vi "TOOLweb ALLE DATEN.vi"(4 "error in (no error)":errorcluster caption="Fehler (Eingang, kein Fehler)", 5 "IP-Adresse (localhost)":string="127.0.0.1", 7 "Anzahl Gase":i32=18) -> (0 "error out":errorcluster caption="Fehler (Ausgang)", 1 "Diagnose":T1, 2 "Info":T3, 3 "Signalverläufe":T2)   [LabVIEW 2020, in "FT-IR.lvlib" / "TOOLweb Interface.lvlib"]
doc: "Holt mit einer HTTP-POST-Anforderung gemäß TOOLweb-Protokoll Messdaten, Einstellungen und Diagnose-Information vom MKS MultiGas 2030 Analyzer. Alle Daten werden zeitsparend in einem einzigen Poll Request zusammengefasst, damit nur einmal eine TCP/IP-Verbindung geöffnet werden muss.\n\nAlle Ergebnis-Datentypen sind als Typdefinitionen in der Bibliothek \"Datentypen\" enthalten\" und erlauben so eine spätere Erweiterung.\n\nFalls \"Anzahl Gase\" unverbunden bleibt, wird der Standardwert 18 verwendet.\n \nFalls der TOOLWeb-Server nicht auf demselben Rechner arbeitet, kann mit \"IP-Adresse\" eine beliebiger Host adressiert werden. Ein unverbundener Eingang spricht den lokalen Host an."
uses:
  TOOLweb Interface.lvlib
  TOOLweb Interface Hilfs-VIs.lvlib
  TOOLweb Info.ctl
  Typdefinitionen.lvlib
  TOOLweb Diagnose.ctl
  TOOLweb Signalverlaeufe.ctl
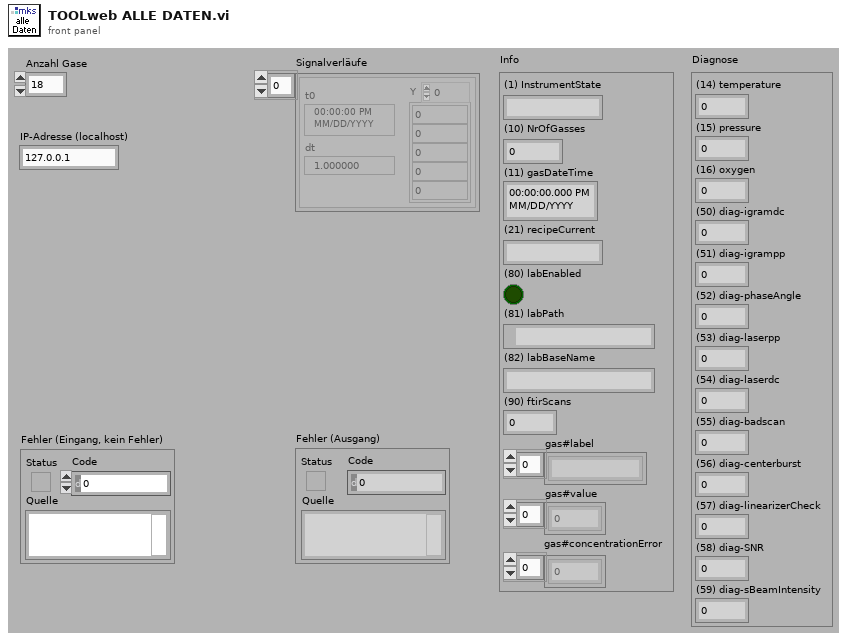
[diagram p1: front panel]
types:
  T1 = typedef "FT-IR.lvlib/TOOLweb Interface.lvlib/Typdefinitionen.lvlib/TOOLweb Diagnose.ctl" = cluster{"(14) temperature":sgl, "(15) pressure":sgl, "(16) oxygen":sgl, "(50) diag-igramdc":sgl, "(51) diag-igrampp":sgl, "(52) diag-phaseAngle":sgl, "(53) diag-laserpp":sgl, "(54) diag-laserdc":sgl, "(55) diag-badscan":sgl, "(56) diag-centerburst":sgl, "(57) diag-linearizerCheck":sgl, "(58) diag-SNR":sgl, "(59) diag-sBeamIntensity":sgl}
  T2 = typedef "FT-IR.lvlib/TOOLweb Interface.lvlib/Typdefinitionen.lvlib/TOOLweb Signalverlaeufe.ctl" = waveform(dbl)[]
  T3 = typedef "FT-IR.lvlib/TOOLweb Interface.lvlib/Typdefinitionen.lvlib/TOOLweb Info.ctl" = cluster{"(1) InstrumentState":string, "(10) NrOfGasses":i32, "(11) gasDateTime":timestamp, "(21) recipeCurrent":string, "(80) labEnabled":bool, "(81) labPath":path, "(82) labBaseName":string, "(90) ftirScans":i32, "gas#label":string[], "gas#value":dbl[], "gas#concentrationError":dbl[]}
  T4 = cluster{"(1) InstrumentState":string, "(10) NrOfGasses":dbl, "(11) gasDateTime":timestamp, "(21) recipeCurrent":string, "(80) labEnabled":bool, "(81) labPath":path, "(82) labBaseName":string, "(90) ftirScans":i32, "gas#label":string[], "gas#value":dbl[], "gas#concentrationError":dbl[]}
  T5 = cluster{"(14) temperature":dbl, "(15) pressure":dbl, "(16) oxygen":dbl, "(50) diag-igramdc":dbl, "(51) diag-igrampp":dbl, "(52) diag-phaseAngle":dbl, "(53) diag-laserpp":dbl, "(54) diag-laserdc":dbl, "(55) diag-badscan":dbl, "(56) diag-centerburst":dbl, "(57) diag-linearizerCheck":dbl, "(58) diag-SNR":dbl, "(59) diag-sBeamIntensity":dbl}
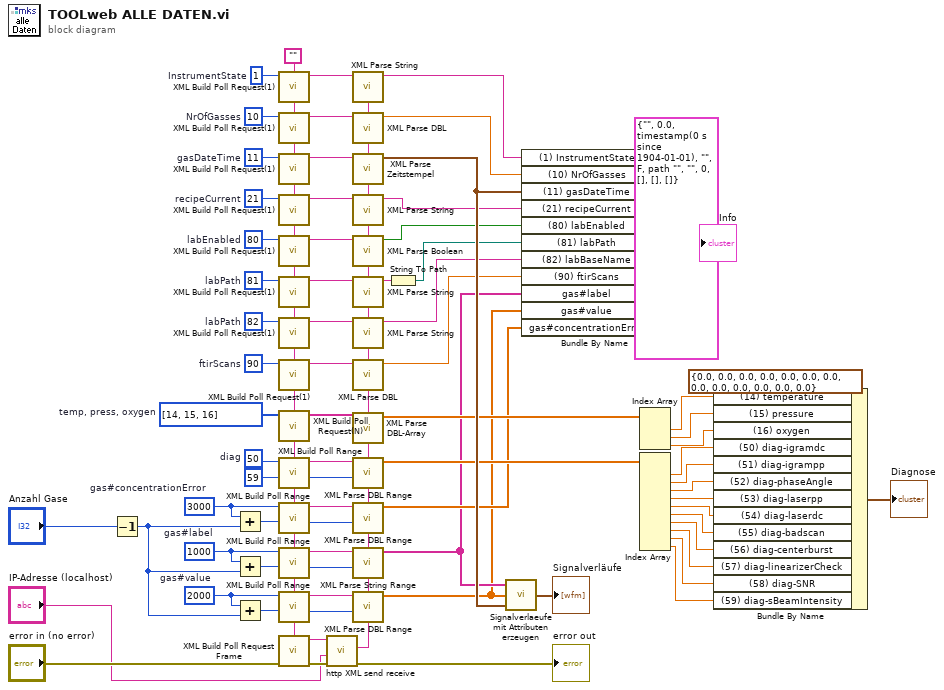
[diagram p0: block diagram]
diagram:
  w33 = 90  # ftirScans
  w37 = 82  # labPath
  w43 = 81  # labPath
  w61 = 50  # diag
  w74 = 1  # InstrumentState
  w76 = 3000  # gas#concentrationError
  w88 = i32[] [14, 15, 16]  # temp, press, oxygen
  w92 = 80  # labEnabled
  w93 = 21  # recipeCurrent
  w94 = 10  # NrOfGasses
  w97 = 2000  # gas#value
  w98 = 1000  # gas#label
  w99 = 11  # gasDateTime
  n1 = Decrement(x="Anzahl Gase") -> (x-1=w75:i32)
  n2 = Add(x=w76, y=w75) -> (x+y=w77:i32)
  n3 = Add(x=w98, y=w75) -> (x+y=w90:i32)
  n4 = Add(x=w97, y=w75) -> (x+y=w89:i32)
  n5 = call "XML Build Poll Request(1).vi"("XML-Message alt"="", "EVID-Nummer"=w74) -> ("Attribut Name"=w72:string, "XML-Message neu"=w15:string)  [unwired: 6 out]
  n6 = call "XML Build Poll Request(1).vi"("XML-Message alt"=w15, "EVID-Nummer"=w94) -> ("Attribut Name"=w95:string, "XML-Message neu"=w29:string)  [unwired: 6 out]
  n7 = call "XML Build Poll Request(1).vi"("XML-Message alt"=w29, "EVID-Nummer"=w99) -> ("Attribut Name"=w96:string, "XML-Message neu"=w5:string)  [unwired: 6 out]
  n8 = call "XML Build Poll Request(1).vi"("XML-Message alt"=w5, "EVID-Nummer"=w93) -> ("Attribut Name"=w91:string, "XML-Message neu"=w4:string)  [unwired: 6 out]
  n9 = call "XML Build Poll Request(1).vi"("XML-Message alt"=w4, "EVID-Nummer"=w92) -> ("Attribut Name"=w67:string, "XML-Message neu"=w28:string)  [unwired: 6 out]
  n10 = call "XML Build Poll Request(1).vi"("XML-Message alt"=w28, "EVID-Nummer"=w43) -> ("Attribut Name"=w41:string, "XML-Message neu"=w38:string)  [unwired: 6 out]
  n11 = call "XML Build Poll Request(1).vi"("XML-Message alt"=w38, "EVID-Nummer"=w37) -> ("Attribut Name"=w35:string, "XML-Message neu"=w27:string)  [unwired: 6 out]
  n12 = call "XML Build Poll Request(1).vi"("XML-Message alt"=w27, "EVID-Nummer"=w33) -> ("Attribut Name"=w32:string, "XML-Message neu"=w14:string)  [unwired: 6 out]
  n13 = call "XML Build Poll Request(N).vi"("XML-Message alt"=w14, "EVID-Nummern"=w88) -> ("Attribut Name (N)"=w66:string[], "XML-Message neu"=w26:string)  [unwired: 6 out]
  n14 = call "XML Build Poll Range.vi"("XML-Message alt"=w26, "von EVID-Nr"=w61, "bis EVID-Nr"=59) -> ("Attribut Name (Range)"=w59:string, "Anzahl Elemente"=w58:i32, "XML-Message neu"=w13:string)  [unwired: 1 in, 3 out]
  n15 = call "XML Build Poll Range.vi"("XML-Message alt"=w13, "von EVID-Nr"=w76, "bis EVID-Nr"=w77) -> ("Attribut Name (Range)"=w78:string, "Anzahl Elemente"=w79:i32, "XML-Message neu"=w25:string)  [unwired: 1 in, 3 out]
  n16 = call "XML Build Poll Range.vi"("XML-Message alt"=w25, "von EVID-Nr"=w98, "bis EVID-Nr"=w90) -> ("Attribut Name (Range)"=w87:string, "Anzahl Elemente"=w86:i32, "XML-Message neu"=w24:string)  [unwired: 1 in, 3 out]
  n17 = call "XML Build Poll Range.vi"("XML-Message alt"=w24, "von EVID-Nr"=w97, "bis EVID-Nr"=w89) -> ("Attribut Name (Range)"=w85:string, "Anzahl Elemente"=w84:i32, "XML-Message neu"=w12:string)  [unwired: 1 in, 3 out]
  n18 = call "XML Build Poll Request Frame.vi"("XML-Message"=w12, "error in (no error)"="error in (no error)") -> ("XML-Message fertig"=w11:string, "error out"=w83:errorcluster)  [unwired: 1 in, 5 out]
  n19 = call "http XML send receive.vi"("error in (no error)"=w83, "IP-Adresse (localhost)"="IP-Adresse (localhost)", "XML Request"=w11) -> ("error out"=→"error out":errorcluster, "Response Body (XML)"=w23:string)  [unwired: 3 out]
  n20 = call "XML Parse DBL Range.vi"("Attribut Name"=w85, "XML Response"=w23, "Anzahl Elemente"=w84) -> ("Werte"=w44:dbl[], "XML Response gekürzt"=w22:string)  [unwired: 5 out]
  n21 = call "XML Parse String Range.vi"("Attribut Name"=w87, "XML Response"=w22, "Anzahl Elemente"=w86) -> ("Elemente (Strings)"=w45:string[], "XML Response gekürzt"=w21:string)  [unwired: 5 out]
  n22 = call "XML Parse DBL Range.vi"("Attribut Name"=w78, "XML Response"=w21, "Anzahl Elemente"=w79) -> ("Werte"=w46:dbl[], "XML Response gekürzt"=w20:string)  [unwired: 5 out]
  n23 = call "XML Parse DBL Range.vi"("Attribut Name"=w59, "XML Response"=w20, "Anzahl Elemente"=w58) -> ("Werte"=w57:dbl[], "XML Response gekürzt"=w19:string)  [unwired: 5 out]
  n24 = call "XML Parse DBL-Array.vi"("Attribut Name"=w66, "XML Response"=w19) -> ("Werte (DBL)"=w65:dbl[], "XML Response gekürzt"=w18:string)  [unwired: 6 out]
  n25 = call "XML Parse DBL.vi"("Attribut Name"=w32, "XML Response"=w18) -> ("Wert (DBL)"=w30:dbl, "XML Response gekürzt"=w31:string)  [unwired: 6 out]
  n26 = call "XML Parse String.vi"("Attribut Name"=w35, "XML Response"=w31) -> ("Wert-String"=w34:string, "XML Response gekürzt"=w36:string)  [unwired: 6 out]
  n27 = call "XML Parse String.vi"("Attribut Name"=w41, "XML Response"=w36) -> ("Wert-String"=w40:string, "XML Response gekürzt"=w42:string)  [unwired: 6 out]
  n28 = call "XML Parse Boolean.vi"("Attribut Name"=w67, "XML Response"=w42) -> ("Wert (boolean)"=w9:bool, "XML Response gekürzt"=w2:string)  [unwired: 6 out]
  n29 = call "XML Parse String.vi"("Attribut Name"=w91, "XML Response"=w2) -> ("Wert-String"=w6:string, "XML Response gekürzt"=w3:string)  [unwired: 6 out]
  n30 = call "XML Parse Zeitstempel.vi"("Attribut Name"=w96, "XML Response"=w3) -> ("Zeitstempel"=w73:timestamp, "XML Response gekürzt"=w17:string)  [unwired: 6 out]
  n31 = call "XML Parse DBL.vi"("Attribut Name"=w95, "XML Response"=w17) -> ("Wert (DBL)"=w69:dbl, "XML Response gekürzt"=w16:string)  [unwired: 6 out]
  n32 = call "XML Parse String.vi"("Attribut Name"=w72, "XML Response"=w16) -> ("Wert-String"=w71:string)  [unwired: 7 out]
  n33 = String To Path(string=w40) -> (path=w39:path)
  n34 = call "Signalverlaeufe mit Attributen erzeugen.vi"("Zeitstempel"=w73, "Messwerte"=w44, "Namen"=w45) -> ("Signalverläufe"=→"Signalverläufe":waveform(dbl)[])
  n35 = Bundle By Name(cluster=T4 {"(1) InstrumentState"="", "(10) NrOfGasses"=0.0, "(11) gasDateTime"=timestamp(0 s since 1904-01-01), "(21) recipeCurrent"="", "(80) labEnabled"=FALSE, "(81) labPath"=path "", "(82) labBaseName"="", "(90) ftirScans"=0, "gas#label"=[], "gas#value"=[], "gas#concentrationError"=[]} ("Info"), "(1) InstrumentState"=w71, "(10) NrOfGasses"=w69, "(11) gasDateTime"=w73, "(21) recipeCurrent"=w6, "(80) labEnabled"=w9, "(81) labPath"=w39, "(82) labBaseName"=w34, "(90) ftirScans"=w30, "gas#label"=w45, "gas#value"=w44, "gas#concentrationError"=w46) -> (→"Info":T4)
  n36 = Index Array(array=w65) -> (element #1=w64:dbl, element #2=w63:dbl, element #3=w62:dbl)  [unwired: 3 in]
  n37 = Index Array(array=w57) -> (element #1=w56:dbl, element #2=w55:dbl, element #3=w54:dbl, element #4=w53:dbl, element #5=w52:dbl, element #6=w51:dbl, element #7=w50:dbl, element #8=w49:dbl, element #9=w48:dbl, element #10=w47:dbl)  [unwired: 10 in]
  n38 = Bundle By Name(cluster=T5 {"(14) temperature"=0.0, "(15) pressure"=0.0, "(16) oxygen"=0.0, "(50) diag-igramdc"=0.0, "(51) diag-igrampp"=0.0, "(52) diag-phaseAngle"=0.0, "(53) diag-laserpp"=0.0, "(54) diag-laserdc"=0.0, "(55) diag-badscan"=0.0, "(56) diag-centerburst"=0.0, "(57) diag-linearizerCheck"=0.0, "(58) diag-SNR"=0.0, "(59) diag-sBeamIntensity"=0.0} ("Diagnose"), "(14) temperature"=w64, "(15) pressure"=w63, "(16) oxygen"=w62, "(50) diag-igramdc"=w56, "(51) diag-igrampp"=w55, "(52) diag-phaseAngle"=w54, "(53) diag-laserpp"=w53, "(54) diag-laserdc"=w52, "(55) diag-badscan"=w51, "(56) diag-centerburst"=w50, "(57) diag-linearizerCheck"=w49, "(58) diag-SNR"=w48, "(59) diag-sBeamIntensity"=w47) -> (→"Diagnose":T5)
